vi "q5 complex number.vi"() -> ()   [LabVIEW 2025]
panel:
  out "Phase \nAngle":dbl
  out "Magnitude":dbl
  in  "Complex \nNumber":cdb
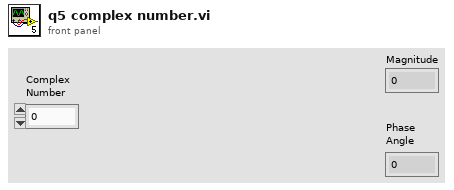
[diagram p1: front panel]
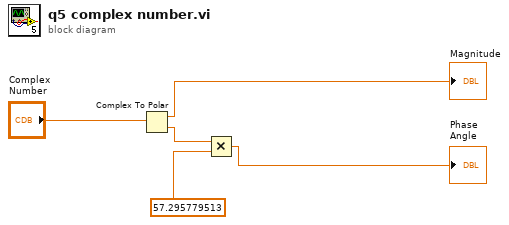
[diagram p0: block diagram]
diagram:
  n1 = Complex To Polar(r * e^(i*theta)="Complex \nNumber") -> (r=→"Magnitude":dbl, theta=w2:dbl)
  n2 = Multiply(x=w2, y=57.295779513) -> (x*y=→"Phase \nAngle":dbl)
